vi "Write Expected result.vi"(8 "error in (no error)":errorcluster, 10 "Expected result":bool, 11 "[Test Case] File or directory exists in":refnum<class "[Test Case] File or directory exists.lvclass">=refnum) -> (0 "error out":errorcluster, 3 "[Test Case] File or directory exists out":refnum<class "[Test Case] File or directory exists.lvclass">)   [LabVIEW 2016, in "Tests.lvlib" / "[Test Case] File or directory exists.lvclass"]
uses:
  [Test Case] File or directory exists.lvclass
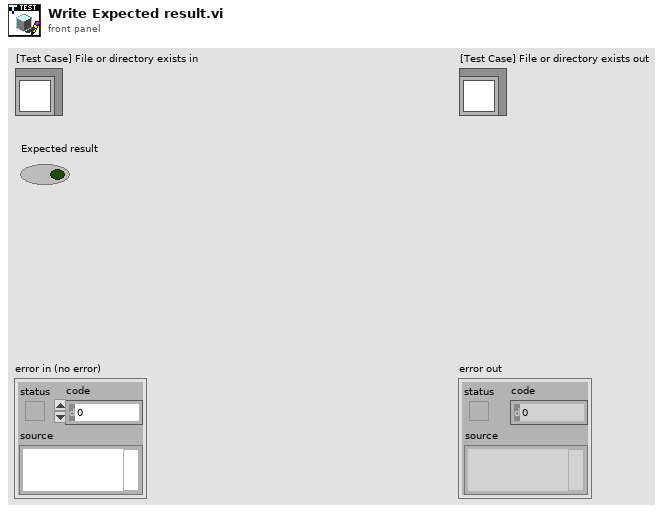
[diagram p1: front panel]
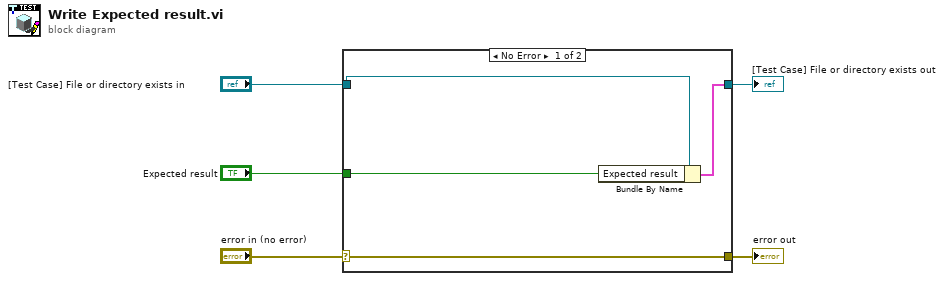
[diagram p0: block diagram]
diagram:
  n1 = case shown="No Error" "error in (no error)" {
    selector: "error in (no error)" -> [w9 w10]
    tunnel: [w9 w10] -> w4
    tunnel: [w7 w11] -> w2
    tunnel: "[Test Case] File or directory exists in" -> [w8 w11]
    tunnel: "Expected result" -> [w6 _]
    frame No Error {
      n2 = Bundle By Name(cluster=w8, "Expected result"=w6) -> (w7:cluster{})
    }
    frame Error {
    }
  }
  "error out" <- w4
  "[Test Case] File or directory exists out" <- w2
